vi "CRYReplace Acquisition Curve Name.vi"(6 "Calibration in":string, 7 "Setup in":T3={"No.VI"=0, "Category"="", "StepName"="", "Seq setup flattened"="", "Comment"="", "Steps config."=[], "Jump config"=[], "Start"=0.0, "Increment"=0.0, "Name"="Pa", "Unit"="Pa", "Y data"=1, "Y prefix"="", "Y dB ref"=1.0, "Y unit"="", "Repeat State Array"=[]} {"Repeat State Array"."Start" format="%#_5g"; "Y dB ref" format="%.1f"; "Y data" items=["dB", "Lin"]; "Start" format="%#_5g"}, 8 "Hardware Setup In":string, 9 "Step Setup In":string, 10 "No Insert CurveLib?":bool, 11 "Type In":string) -> (0 "Current Name Out":string[][](array[string]), 2 "Waves Out":T2 {"Y dB ref" format="%.1f"; "Y axis" items=["Log", "Lin"]; "Y data" items=["dB", "Lin"]; "X data" items=["dB", "Lin"]}, 3 "Inserted Names Out":string[](array[string]))   [LabVIEW 2013]
uses:
  Typedef Control/CRYData Variant Array.ctl
  Typedef Control/CRYWaveform Cluster.ctl
  Typedef Control/CRYData Cluster.ctl
  Typedef Control/CRYStep.ctl
  Typedef Control/CRYWaveform Cluster Array.ctl
  Calibration/SubVI/CRYCal Global.vi
panel:
  out "Index for testinfor":i32
  in  "Waveform Cluster":T1={"Waveform"={"X0"=0.0, "dX"=0.0, "Y"=[]}, "X data"=1, "Y data"=1, "Y axis"=1, "X unit"="s", "Y unit"="V", "Y dB ref"=1.0, "display Y"=TRUE, "display X"=TRUE, "Overload?"=FALSE, "Test Info"="", "Step No."=0, "Name"="", "protected"=FALSE, "Sqc history"=[], "Signal Channel ID"=0, "Plot Settings"={"Color"=0, "Interpolation"=0, "Point Style"=0, "Line Style"=0, "Point Color"=0, "Line Width"=0, "Bar Plot Style"=0, "Fill To"=0}, "AutoProtect"=FALSE} {"Y dB ref" format="%.1f"; "Y axis" items=["Log", "Lin"]; "Y data" items=["dB", "Lin"]; "X data" items=["dB", "Lin"]}
  in  "Data In":T4[](array[typedef]) {"Z data" items=["dB", "Lin"]; "X data" items=["dB", "Lin"]; "Y data" items=["dB", "Lin"]; "Z dB ref" format="%.1f"; "Z axis" items=["Log", "Lin"]; "X dB ref" format="%.1f"; "X axis" items=["Log", "Lin"]; "Y axis" items=["Log", "Lin"]; "Y dB ref" format="%.1f"; "Curve"."z" format="%.2f"; "Curve"."y" format="%.2f"; "Curve"."x" format="%.2f"}
  in  "Wave In":T1[](array[typedef]) {"Y dB ref" format="%.1f"; "Y axis" items=["Log", "Lin"]; "Y data" items=["dB", "Lin"]; "X data" items=["dB", "Lin"]}
  in  "Data":T5
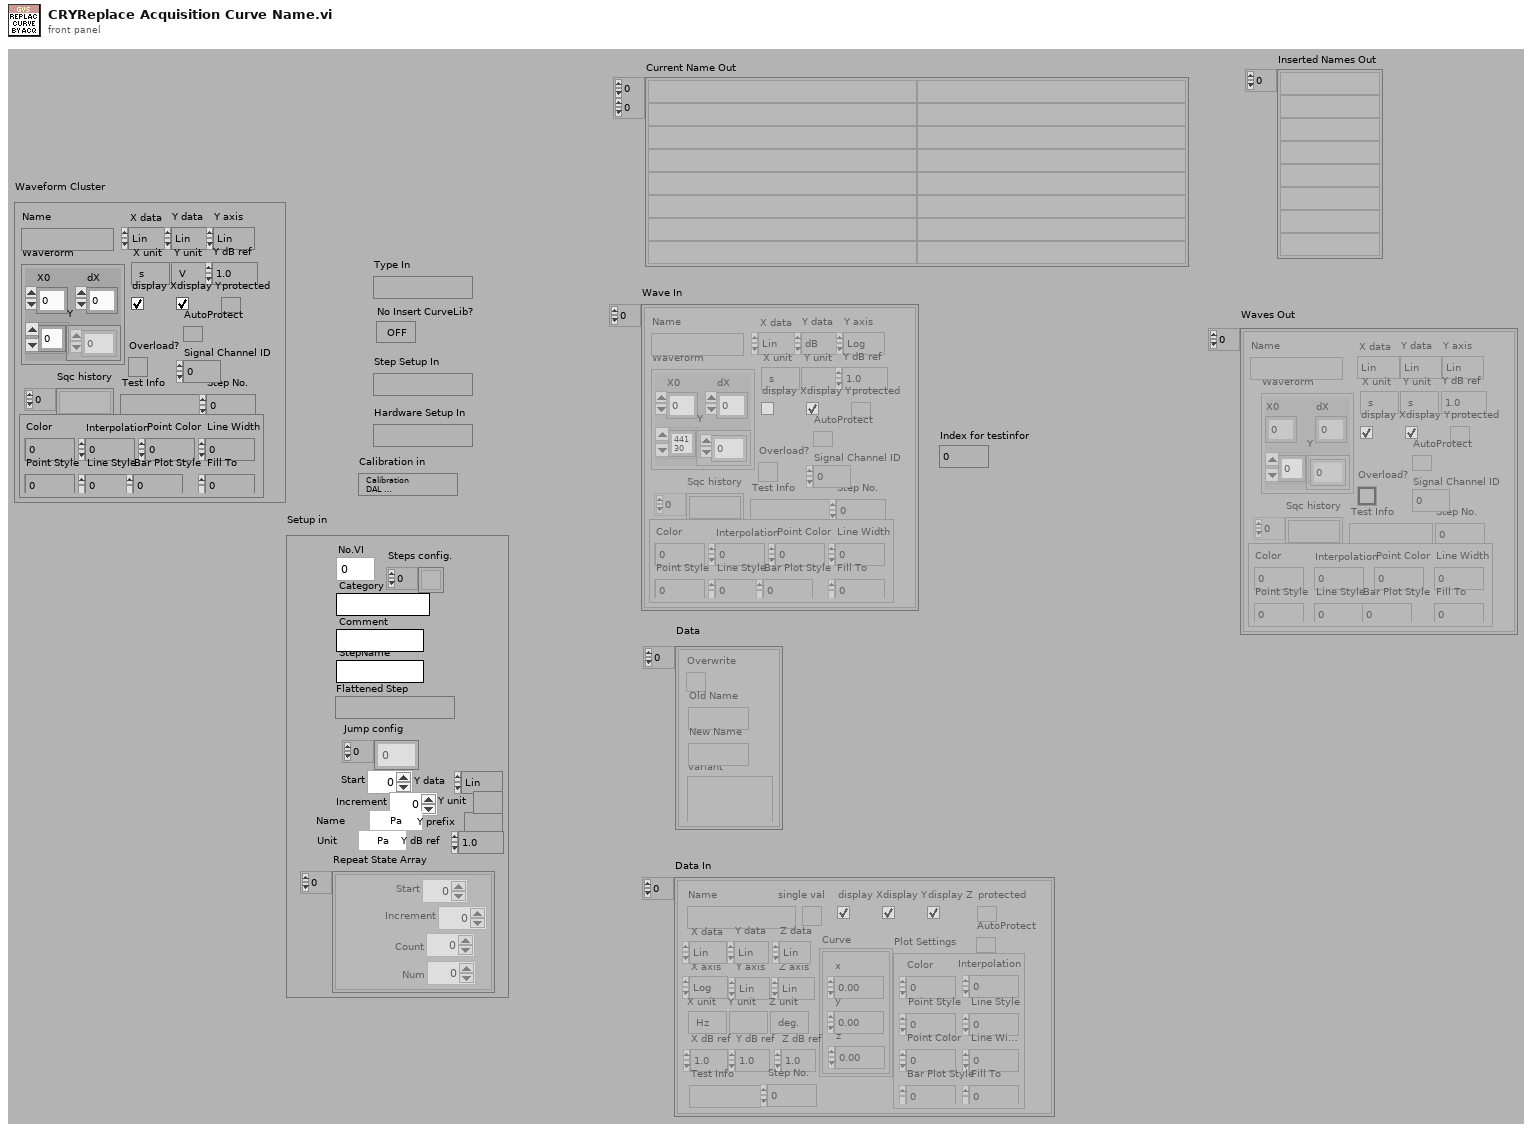
[diagram p1: front panel]
types:
  T1 = typedef "CRYWaveform Cluster.ctl" = cluster{"Waveform":cluster{"X0":dbl, "dX":dbl, "Y":sgl[]}, "X data":u16, "Y data":u16, "Y axis":u16, "X unit":string, "Y unit":string, "Y dB ref":dbl, "display Y":bool, "display X":bool, "Overload?":bool, "Test Info":string, "Step No.":i32, "Name":string, "protected":bool, "Sqc history":string[], "Signal Channel ID":i32, "Plot Settings":cluster{"Color":u32, "Interpolation":u8, "Point Style":u8, "Line Style":u8, "Point Color":u32, "Line Width":u8, "Bar Plot Style":u8, "Fill To":i16}, "AutoProtect":bool}
  T2 = typedef "CRYWaveform Cluster Array.ctl" = T1[]
  T3 = typedef "CRYStep.ctl" = cluster{"No.VI":i32, "Category":string, "StepName":string, "Seq setup flattened":string, "Comment":string, "Steps config.":bool[], "Jump config":i32[], "Start":dbl, "Increment":dbl, "Name":string, "Unit":string, "Y data":u16, "Y prefix":string, "Y dB ref":dbl, "Y unit":string, "Repeat State Array":cluster{"Start":dbl, "Increment":dbl, "Count":i32, "Num":i32}[]}
  T4 = typedef "CRYData Cluster.ctl" = cluster{"Name":string, "Curve":cluster{"x":dbl, "y":dbl, "z":dbl}[], "X data":u16, "Y data":u16, "Z data":u16, "X axis":u16, "Y axis":u16, "Z axis":u16, "X unit":string, "Y unit":string, "Z unit":string, "X dB ref":dbl, "Y dB ref":dbl, "Z dB ref":dbl, "single val":bool, "protected":bool, "display X":bool, "display Y":bool, "display Z":bool, "Test Info":string, "Step No.":i32, "Plot Settings":cluster{"Color":u32, "Interpolation":u8, "Point Style":u8, "Line Style":u8, "Point Color":u32, "Line Width":u8, "Bar Plot Style":u8, "Fill To":i16}, "AutoProtect":bool}
  T5 = typedef "CRYData Variant Array.ctl" = cluster{"variant":variant, "Overwrite":bool, "Old Name":string, "New Name":string}[]
  T6 = enum16{"Play & Record", "Record", "Sine Generator", "Voltmeter", "Oscilloscope", "Spectrum Analyzer", "RTA", "Generator & Voltmeter", "Generator & Oscilloscope", "Generator & Spectrum", "Generator & RTA"}
  T7 = typedef "CRYAcquisition Cluster.ctl" = cluster{"Mode":u16, "Name":string, "use ch name":bool, "Record Time":dbl, "hide rec":bool, "hide play":bool, "rec delay":dbl, "rec pad":dbl, "dcc units":i8, "sine gen setting":string, "scope_fft setting":string, "voltmeter setting":string, "rta setting":string, "trig offset(sec)":dbl, "triggered  record":bool, "trig level":dbl, "trig unit":u8, "trig slop":bool, "trig timeout(sec)":dbl, "add record":bool, "EQ":bool, "record table":string[][], "play table":string[][], "trig channel":string, "Help":string}
  T8 = cluster{"Start":dbl, "Increment":dbl, "Count":i32, "Num":i32}[]
  T9 = typedef "CRYCalibration 2DCluster.ctl" = cluster{"Calibration":T10, "Corr Curve":T4, "EQ Curve":T4, "Sens Curve":T4}
  T10 = typedef "CRYCalibration Cluster.ctl" = cluster{"Calibration Step Name":string, "Device":string, "Correction Curve Name":string, "Equalization Curve Name":string, "Sensitivity Curve Name":string, "Corr Folder and File":string, "EQ Folder and File":string, "Sens Folder and File":string, "Corr Step size":u16, "EQ Step size":u16, "Input":bool, "Last Cal Date (sec)":timestamp, "Cha Name":string, "Corr Curve Found":bool, "EQ Curve Found":bool, "Sens Curve Found":bool, "Signal Type":string, "Calibrated Device":string, "Hz":u32}
  T11 = typedef "CRYCalibration All Cluster.ctl" = cluster{"Calibration 2D":T9[], "Help":string, "Tab Value":i32, "Input Signal Type":string, "Output Signal Type":string}
  T12 = typedef "CRYHardware Channel Info.ctl" = cluster{"ID":i32, "Name":string, "Digital":bool, "Input":bool, "Device Name":string, "Hardware Ch ID":u8, "Vmax (V)":dbl, "Latency (samples)":dbl, "Sampling Rate (Hz)":u32, "Bit Depth":u32, "Anti-aliasing Factor (%fs)":sgl, "DAQmx Channel":tag, "term config":i32, "Coupling":i32, "IEPE en":bool, "ASIOChannel Name":string, "Audio Driver":u16, "ASIOChannel Index":u8}
  T13 = cluster{"MME Record Cluster":cluster{"RecDeviceID":u32, "RecSampleFreq":u32, "RecChannels":u32, "RecBitDepth":u32, "RecSampleData":i32[], "RecDataLength":u32, "RecTime":sgl, "RecLatency":sgl, "RecPadding":sgl, "nBufferUse":u32, "nRealTime":u32, "Anti Alias":u32, "Device Name":string, "Audio Driver":u16}[], "ASIO Record Cluster":cluster{"RecDeviceID":u32, "RecSampleFreq":u32, "RecChannels":u32, "RecBitDepth":u32, "RecSampleData":i32[], "RecDataLength":u32, "RecTime":sgl, "RecLatency":sgl, "RecPadding":sgl, "nBufferUse":u32, "nRealTime":u32, "Anti Alias":u32, "Device Name":string, "Audio Driver":u16}[]}
  T14 = cluster{"RecDeviceID":u32, "RecSampleFreq":u32, "RecChannels":u32, "RecBitDepth":u32, "RecSampleData":i32[], "RecDataLength":u32, "RecTime":sgl, "RecLatency":sgl, "RecPadding":sgl, "nBufferUse":u32, "nRealTime":u32, "Anti Alias":u32, "Device Name":string, "Audio Driver":u16}[]
  T15 = typedef "CRYStimulus Test Infor Cluster.ctl" = cluster{"Stimulus Type":string, "Signal Type":string, "In/Out":bool, "FAPS":cluster{"freq":dbl, "ampl":dbl, "cycles":dbl, "samples":i32}[], "Sampling Rate":dbl, "Samples":i32, "Analysis Param":string, "Resolution":u16, "Steps":u32, "Analysis Value":dbl[], "Diff Freq":dbl, "FStart":dbl, "FStop":dbl, "Calibration Param":string, "Anti Alias":dbl, "Level Out1":dbl, "Level Out2":dbl, "EQ":bool}
  T16 = typedef "CRYData Cluster Array.ctl" = T4[]
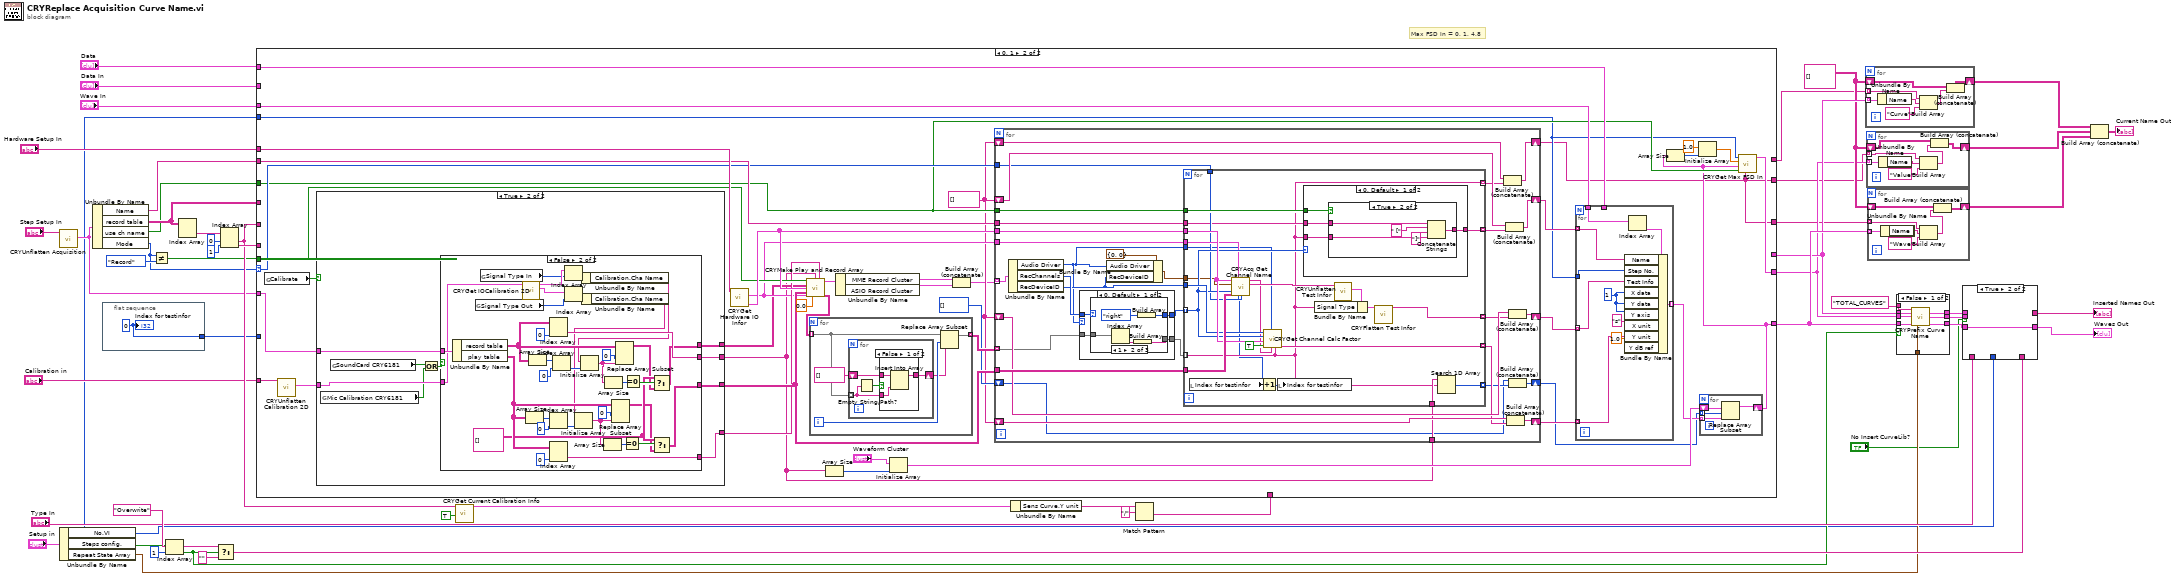
[diagram p0: block diagram]
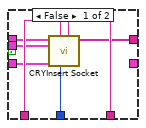
[diagram p2: hidden frame]
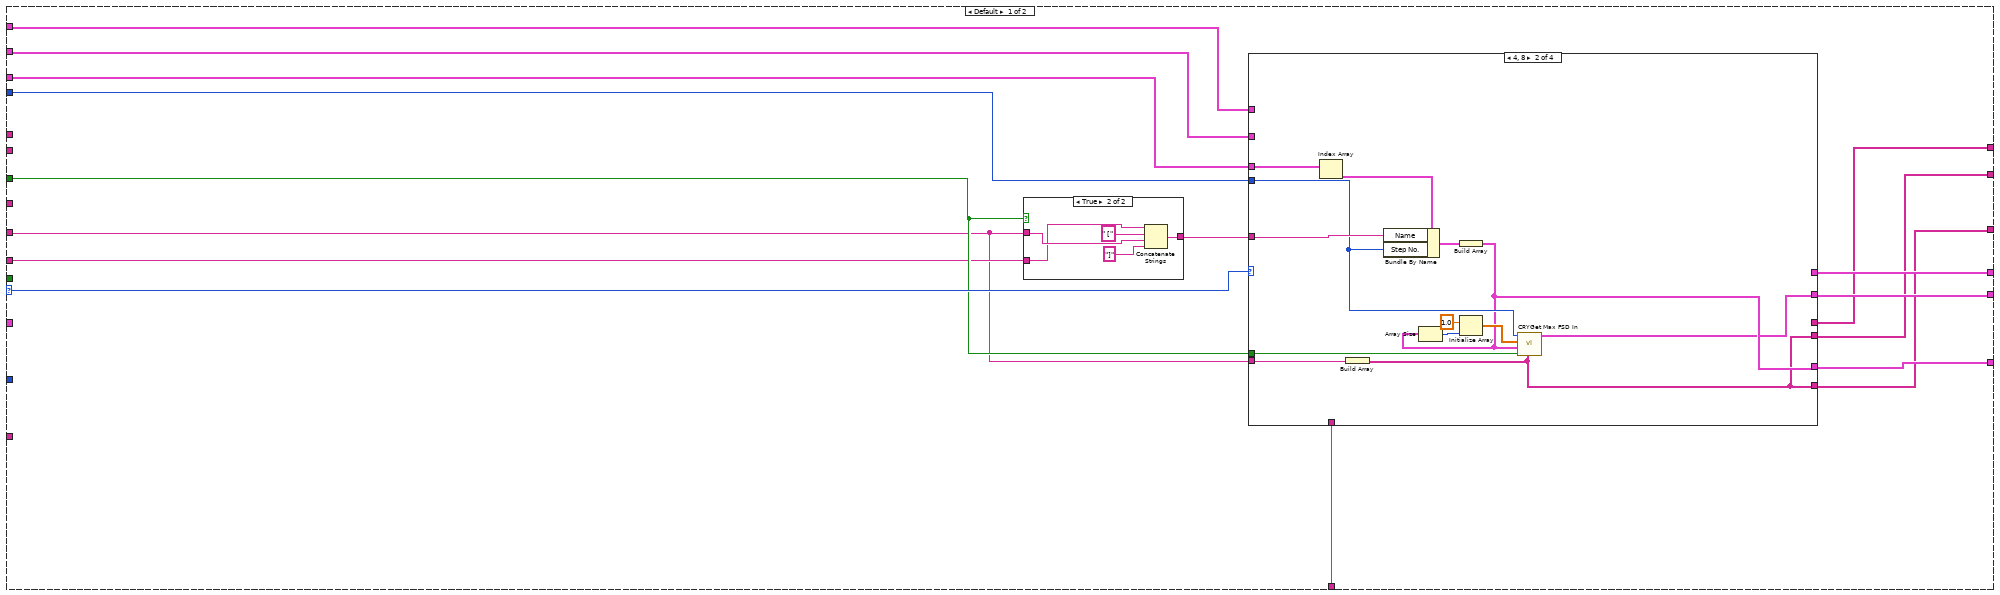
[diagram p4: hidden frame]
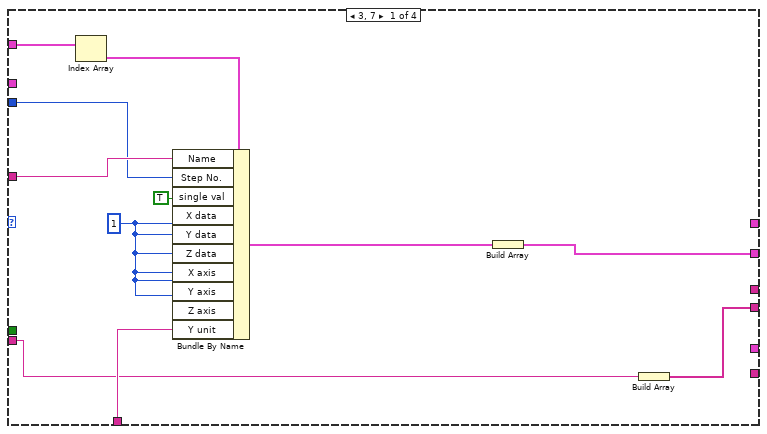
[diagram p5: hidden frame]
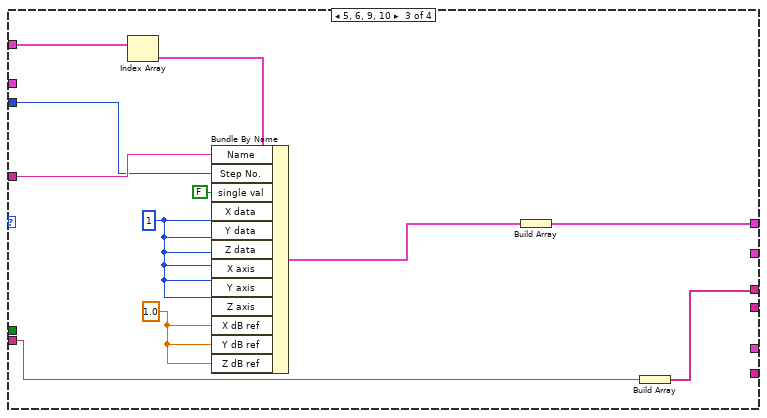
[diagram p6: hidden frame]
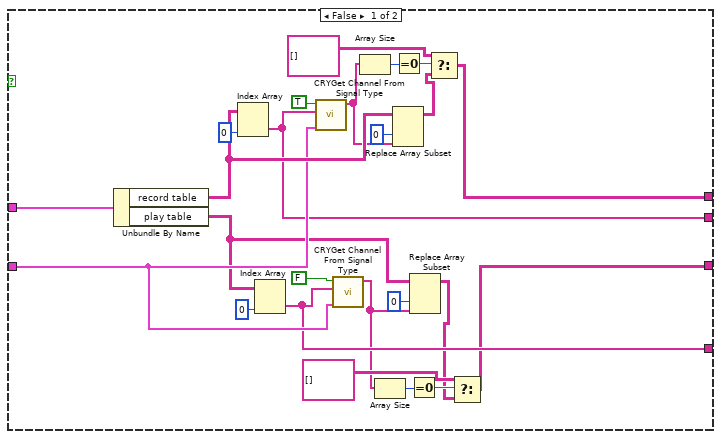
[diagram p10: hidden frame]
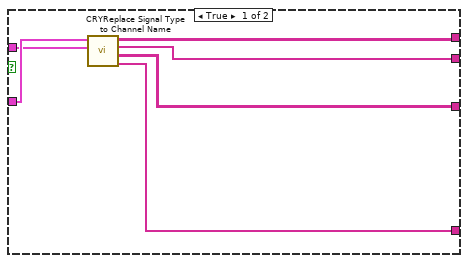
[diagram p11: hidden frame]
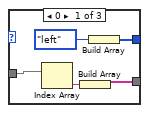
[diagram p12: hidden frame]
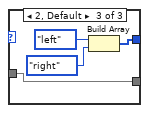
[diagram p13: hidden frame]
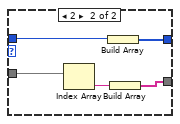
[diagram p14: hidden frame]
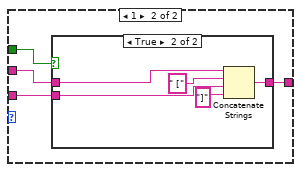
[diagram p16: hidden frame]
diagram:
  w11 = string[][] []
  # "Max FSD In = 0, 1, 4,8"
  n1 = call "CRYUnflatten Acquisition.vi"("Flatten Acquisition"="Step Setup In") -> ("Acquisition"=w17:T7)  [unwired: 10 out]
  n2 = Unbundle By Name("Setup in") -> ("No.VI"=w14:i32, "Steps config."=w33:bool[], "Repeat State Array"=w24:T8)
  n3 = Unbundle By Name(w17) -> ("Name"=w16:string, "record table"=w20:string[][], "use ch name"=w10:bool, "Mode"=w15:u16)
  n4 = flat-sequence {
    tunnel: [w53] -> w1
    frame #0 {
      w53 = 0 ("Index for testinfor")
      "Index for testinfor" <- w53
    }
  }
  n5 = Not Equal?(x=w15, y=T6."Record" ("Record Mode")) -> (x != y?=w19:bool)
  n6 = Index Array(array=w33, index=1) -> (element=w25:bool)
  n7 = Index Array(array=w20) -> (element=w48:string[])  [unwired: 2 in]
  n8 = Select(t="Overwrite" ("Y unit"), s=w25, f="") -> (s? t:f=w31:string)
  n9 = Index Array(array=w48, index #1=0 ("index"), index #2=1 ("index")) -> (element #1=w39:string, element #2=w47:string)
  n10 = call "CRYGet Current Calibration Info.vi"("Is Input?"=TRUE, "Signal Type Name"=w39) -> ("Calibration All Cluster"=w42:T9)  [unwired: 9 out]
  n11 = Unbundle By Name(w42) -> ("Sens Curve.Y unit"=w40:string)
  n12 = Match Pattern(string=w40, regular expression="/" ("search char (-)")) -> (after substring=w38:string)  [unwired: 4 out]
  n13 = case shown="0, 1" w15 {
    selector: w15 -> [w64 w134]
    tunnel: w47 -> [w58 _]
    tunnel: w10 -> [w59 w120]
    tunnel: w39 -> [w57 _]
    tunnel: "Data" -> [w68 w149]
    tunnel: "Wave In" -> [w67 w148]
    tunnel: w14 -> [w65 w118]
    tunnel: "Data In" -> [w69 _]
    tunnel: w38 -> [w63 _]
    tunnel: [w61 w117] -> w13
    tunnel: [w62 w119] -> w9
    tunnel: [w60 _] -> w12
    tunnel: "Hardware Setup In" -> [_ w145]
    tunnel: w20 -> [_ _]
    tunnel: w19 -> [_ w143]
    tunnel: "Calibration in" -> [_ w141]
    tunnel: w17 -> [_ w140]
    tunnel: w16 -> [_ w135]
    tunnel: [w54 w115] -> w4
    tunnel: [w56 w115] -> w3
    tunnel: [w55 _] -> w2
    tunnel: w1 -> [_ _]
    frame Default {
      n14 = case shown="True" w59 {
        tunnel: w57 -> [_ w108]
        tunnel: [w105 w107] -> w66
        tunnel: w58 -> [w105 w106]
        frame False {
        }
        frame True {
          n15 = Concatenate Strings(w106, " [" ("string"), w108, "]" ("string")) -> (w107:string)
        }
      }
      n16 = case shown="4, 8" w64 {
        tunnel: w67 -> [_ w93 _ _]
        tunnel: w68 -> [_ _ _ _]
        tunnel: w69 -> [w80 _ w104 _]
        tunnel: w66 -> [w78 w91 w102 _]
        tunnel: w65 -> [w74 w85 w98 _]
        tunnel: w63 -> [w75 _ _ _]
        tunnel: [w72 w83 _ _] -> w62
        tunnel: [_ w84 _ _] -> w61
        tunnel: [_ _ w96 _] -> w60
        tunnel: w59 -> [_ w86 _ _]
        tunnel: w57 -> [w71 w82 w95 _]
        tunnel: [_ w81 _ _] -> w56
        tunnel: [_ _ w94 _] -> w55
        tunnel: [w70 w81 _ _] -> w54
        frame 3, 7 {
          w76 = u16 1 ("X data")
          n17 = Index Array(array=w80) -> (element=w79:T4)  [unwired: 1 in]
          n18 = Bundle By Name(cluster=w79, "Name"=w78, "Step No."=w74, "single val"=TRUE, "X data"=w76, "Y data"=w76, "Z data"=w76, "X axis"=w76, "Y axis"=w76, "Z axis"=w76, "Y unit"=w75) -> (w73:T4)
          n19 = Build Array(w73) -> (w72:T4[])
          n20 = Build Array(w71) -> (w70:string[])
        }
        frame 4, 8 {
          n21 = Index Array(array=w93) -> (element=w92:T1)  [unwired: 1 in]
          n22 = Build Array(w82) -> (w81:string[])
          n23 = Bundle By Name(cluster=w92, "Name"=w91, "Step No."=w85) -> (w90:T1)
          n24 = Build Array(w90) -> (w84:T1[])
          n25 = Array Size(array=w84) -> (size(s)=w87:i32)
          n26 = Initialize Array(1.0 ("element"), w87) -> (w89:dbl[])
          n27 = call "CRYGet Max FSD In.vi"("Signal Path"=w81, "use ch name"=w86, "Wave in"=w84, "Max Level"=w89, "Step No."=w85) -> ("Data Out"=w83:T4[])  [unwired: 6 in]
        }
        frame 5, 6, 9, 10 {
          w99 = 1.0 ("X dB ref")
          w100 = u16 1 ("X data")
          n28 = Index Array(array=w104) -> (element=w103:T4)  [unwired: 1 in]
          n29 = Bundle By Name(cluster=w103, "Name"=w102, "Step No."=w98, "single val"=FALSE, "X data"=w100, "Y data"=w100, "Z data"=w100, "X axis"=w100, "Y axis"=w100, "Z axis"=w100, "X dB ref"=w99, "Y dB ref"=w99, "Z dB ref"=w99) -> (w97:T4)
          n30 = Build Array(w97) -> (w96:T4[])
          n31 = Build Array(w95) -> (w94:string[])
        }
        frame Default {
        }
      }
    }
    frame 0, 1 {
      w116 = string[] [] ("appended array")
      n32 = global read "CRYCal Global.vi" "Calibrate"() -> (w139:bool)
      n33 = call "CRYUnflatten Calibration 2D.vi"("Flattened Calibration"=w141) -> ("Calibration Step Out"=w142:T11)  [unwired: 8 in, 2 out]
      n34 = case shown="True" w139 {
        tunnel: [w175 w197] -> w130
        tunnel: [w169 w196] -> w138
        tunnel: w140 -> [w192 w201]
        tunnel: w142 -> [w184 w198]
        tunnel: [w182 w200] -> w137
        tunnel: [w181 w199] -> w126
        frame False {
          n35 = Unbundle By Name(w192) -> ("record table"=w189:string[][], "play table"=w183:string[][])
          n36 = Index Array(array=w189, index (col)=0 ("disabled index (col)")) -> (element=w181:string[])  [unwired: 1 in]
          n37 = Index Array(array=w183, index (col)=0 ("disabled index (col)")) -> (element=w182:string[])  [unwired: 1 in]
          n38 = call "CRYGet Channel From Signal Type.vi"("Calibration"=w184, "Signal Type Name Array In"=w181, "In/Out?"=TRUE) -> ("Channel Name Array Out"=w177:string[])  [unwired: 7 in, 1 out]
          n39 = call "CRYGet Channel From Signal Type.vi"("Calibration"=w184, "Signal Type Name Array In"=w182, "In/Out?"=FALSE) -> ("Channel Name Array Out"=w171:string[])  [unwired: 7 in, 1 out]
          n40 = Array Size(array=w177) -> (size(s)=w178:i32)
          n41 = Array Size(array=w171) -> (size(s)=w174:i32)
          n42 = Replace Array Subset(array=w189, new element=w177, index (col)=0 ("disabled index (col)")) -> (w176:string[][])  [unwired: 1 in]
          n43 = Equal To 0?(x=w178) -> (x = 0?=w179:bool)
          n44 = Equal To 0?(x=w174) -> (x = 0?=w173:bool)
          n45 = Replace Array Subset(array=w183, new element=w171, index (col)=0 ("disabled index (col)")) -> (w170:string[][])  [unwired: 1 in]
          n46 = Select(t=string[][] [] ("output array"), s=w179, f=w176) -> (s? t:f=w175:string[][])
          n47 = Select(t=string[][] [] ("output array"), s=w173, f=w170) -> (s? t:f=w169:string[][])
        }
        frame True {
          n48 = global read "CRYCal Global.vi" "Mic Calibration CRY6181"() -> (w195:bool)
          n49 = global read "CRYCal Global.vi" "SoundCard CRY6181"() -> (w194:bool)
          n50 = Or(x=w194, y=w195) -> (x .or. y?=w193:bool)
          n51 = case shown="False" w193 {
            tunnel: w201 -> [w206 w239]
            tunnel: [w202 w231] -> w200
            tunnel: [w204 w228] -> w199
            tunnel: w198 -> [w207 w227]
            tunnel: [w203 w211] -> w196
            tunnel: [w205 w208] -> w197
            frame True {
              n52 = call "CRYReplace Signal Type to Channel Name.vi"("Acquisition step in"=w206, "Calibration Step in"=w207) -> ("Play Signal Type"=w202:string[], "Play table"=w203:string[][], "Record Signal Type"=w204:string[], "record table"=w205:string[][])  [unwired: 6 in]
            }
            frame False {
              w213 = string[][] [] ("output array")
              n53 = Unbundle By Name(w239) -> ("record table"=w229:string[][], "play table"=w233:string[][])
              n54 = global read "CRYCal Global.vi" "Signal Type Out"() -> (w219:u16)
              n55 = global read "CRYCal Global.vi" "Signal Type In"() -> (w223:u16)
              n56 = call "CRYGet IOCalibration 2D.vi"("Calibration"=w227) -> ("O_Calibration 2D Out"=w220:T9[], "I_Calibration 2D Out"=w224:T9[])  [unwired: 9 in]
              n57 = Array Size(array=w233) -> (size(s)=w234:i32[])
              n58 = Array Size(array=w229) -> (size(s)=w242:i32[])
              n59 = Index Array(array=w229, index (col)=0 ("disabled index (col)")) -> (element=w228:string[])  [unwired: 1 in]
              n60 = Index Array(array=w233, index (col)=0 ("disabled index (col)")) -> (element=w231:string[])  [unwired: 1 in]
              n61 = Index Array(array=w234, index=0) -> (element=w237:i32)
              n62 = Index Array(array=w242, index=0) -> (element=w238:i32)
              n63 = Index Array(array=w224, index=w223) -> (element=w222:T9)
              n64 = Index Array(array=w220, index=w219) -> (element=w221:T9)
              n65 = Unbundle By Name(w222) -> ("Calibration.Cha Name"=w226:string)
              n66 = Initialize Array(w226, w238) -> (w214:string[])
              n67 = Unbundle By Name(w221) -> ("Calibration.Cha Name"=w225:string)
              n68 = Initialize Array(w225, w237) -> (w210:string[])
              n69 = Array Size(array=w210) -> (size(s)=w218:i32)
              n70 = Array Size(array=w214) -> (size(s)=w216:i32)
              n71 = Replace Array Subset(array=w233, new element=w210, index (col)=0 ("disabled index (col)")) -> (w212:string[][])  [unwired: 1 in]
              n72 = Replace Array Subset(array=w229, new element=w214, index (col)=0 ("disabled index (col)")) -> (w209:string[][])  [unwired: 1 in]
              n73 = Equal To 0?(x=w218) -> (x = 0?=w217:bool)
              n74 = Equal To 0?(x=w216) -> (x = 0?=w215:bool)
              n75 = Select(t=w213, s=w215, f=w209) -> (s? t:f=w208:string[][])
              n76 = Select(t=w213, s=w217, f=w212) -> (s? t:f=w211:string[][])
            }
          }
        }
      }
      n77 = call "CRYGet Hardware IO Infor.vi"("Hardware setup In"=w145) -> ("I_channel Info Out"=w144:T12[], "O_channel Info Out"=w136:T12[])  [unwired: 9 out]
      n78 = call "CRYMake Play and Record Array.vi"("Play&Record/Record"=w143, "Selected Record Signal Path In"=w126, "Selected Play Signal Path In"=w137, "Selected Record In"=w130, "input channel Info In"=w144, "Selected Play In"=w138, "output channel Info In"=w136, "Rec Time"=0.0) -> ("Record Cluster Out"=w114:T13, "Record Name Array"=w133:string[][])  [unwired: 2 in, 4 out]
      n79 = for {
        tunnel: w133 -> [w159] mode=indexing
        tunnel: [w158] -> w132 mode=indexing
        i -> [w157]
        n80 = for {
          tunnel: w159 -> [w162] mode=indexing
          shift-right: [w161] -> w156
          shift-left: string[] [] ("Record Name Array") -> [w163]
          n81 = Empty String/Path?(string/path=w162) -> (empty?=w164:bool)
          n82 = case shown="False" w164 {
            tunnel: w163 -> [w167 w168]
            tunnel: w162 -> [w166 _]
            tunnel: [w165 w168] -> w161
            frame False {
              n83 = Insert Into Array(array=w167, new element=w166) -> (w165:string[])  [unwired: 1 in]
            }
            frame True {
            }
          }
        }
        n84 = Replace Array Subset(array=w159, new element=w156, index=w157) -> (w158:string[])
      }
      n85 = Array Size(array=w126) -> (size(s)=w131:i32)
      n86 = Unbundle By Name(w114) -> ("MME Record Cluster"=w113:T14, "ASIO Record Cluster"=w112:T14)
      n87 = Initialize Array("Waveform Cluster", w131) -> (w128:T1[])
      n88 = Build Array (concatenate)(w113, w112) -> (w111:T14)
      n89 = for {
        tunnel: w111 -> [w283] mode=indexing
        tunnel: w144 -> [w280]
        tunnel: w138 -> [w279]
        tunnel: w120 -> [w278]
        tunnel: w135 -> [w277]
        shift-right: [w274] -> w151
        shift-left: w116 -> [w275]
        shift-right: [w271] -> w150
        shift-left: w116 -> [w273]
        shift-right: [w268] -> w147
        shift-left: w116 -> [w270]
        tunnel: w132 -> [w267] mode=indexing
        tunnel: w136 -> [w265]
        tunnel: w134 -> [w264]
        tunnel: w126 -> [w263]
        shift-right: [w261] -> w124
        shift-left: i32[] [] -> [w260]
        shift-right: [w257] -> w115
        shift-left: w116 -> [w258]
        n90 = Unbundle By Name(w283) -> ("Audio Driver"=w253:u16, "RecChannels"=w282:u32, "RecDeviceID"=w255:u32)
        n91 = case shown="0, Default" w253 {
          tunnel: w282 -> [w287 w302]
          tunnel: [w286 w306] -> w281
          tunnel: w267 -> [w285 w305]
          tunnel: [w284 w304] -> w266
          frame 0, Default {
            n92 = case shown="1" w287 {
              tunnel: [w291 w296 w299] -> w286
              tunnel: w285 -> [w289 w294 w298]
              tunnel: [w288 w293 w298] -> w284
              frame 0 {
                n93 = Index Array(array=w289) -> (element=w290:string)  [unwired: 1 in]
                n94 = Build Array(w290) -> (w288:string[])
                n95 = Build Array(enum16{"left", "right"}."left") -> (w291:enum16{"left", "right"}[])
              }
              frame 1 {
                n96 = Index Array(array=w294) -> (element=w295:string)  [unwired: 1 in]
                n97 = Build Array(w295) -> (w293:string[])
                n98 = Build Array(enum16{"left", "right"}."right") -> (w296:enum16{"left", "right"}[])
              }
              frame 2, Default {
                n99 = Build Array(enum16{"left", "right"}."left", enum16{"left", "right"}."right") -> (w299:enum16{"left", "right"}[])
              }
            }
          }
          frame 2 {
            n100 = Index Array(array=w305) -> (element=w303:string)  [unwired: 1 in]
            n101 = Build Array(w302) -> (w306:u32[])
            n102 = Build Array(w303) -> (w304:string[])
          }
        }
        n103 = Bundle By Name(cluster=cluster{"RecDeviceID":u32, "Audio Driver":u32} {"RecDeviceID"=0, "Audio Driver"=0} ("Cluster"), "Audio Driver"=w253, "RecDeviceID"=w255) -> (w254:cluster{"RecDeviceID":u32, "Audio Driver":u32})
        n104 = for {
          tunnel: w281 -> [w320] mode=indexing
          tunnel: w255 -> [w321]
          tunnel: w280 -> [w322]
          tunnel: w279 -> [w329]
          tunnel: w278 -> [w325]
          tunnel: w277 -> [w312]
          tunnel: [w324] -> w276 mode=indexing
          tunnel: [w323] -> w272 mode=indexing
          tunnel: [w318] -> w269 mode=indexing
          tunnel: w266 -> [w311] mode=indexing
          tunnel: w265 -> [w316]
          tunnel: w264 -> [w315]
          tunnel: w263 -> [w314]
          tunnel: [w313] -> w262 mode=indexing
          tunnel: [w311] -> w259 mode=indexing
          tunnel: w254 -> [w310]
          tunnel: w253 -> [w309]
          n105 = local read "Index for testinfor"() -> (w307:i32)
          n106 = call "CRYAcq Get Channel Name.vi"("I_channel Info Out"=w322, "O_channel Info Out"=w316, "Cluster"=w310, "RecChannel"=w320, "Selected Play In"=w329, "Index for testinfor"=w307, "Acquisition Type"=w315) -> ("ChannelName In"=w317:string, "Test Info"=w326:string)  [unwired: 3 in, 4 out]
          n107 = Increment(x=w307) -> (x+1=w308:i32)
          n108 = call "CRYGet Channel Calc Factor.vi"("Signal Path"=w311, "Channel Name"=w317, "Audio Driver"=w309, "Is Input?"=TRUE, "I/O_channel Info"=w322, "Channel(LR)"=w320, "DeviceID"=w321) -> ("Y unit"=w318:string)  [unwired: 4 out]
          n109 = local write "Index for testinfor"(w308) -> ()
          n110 = case shown="0, Default" w320 {
            tunnel: [w332 w342] -> w324
            tunnel: w312 -> [w333 w343]
            tunnel: w311 -> [w331 w341]
            tunnel: w325 -> [w330 w340]
            frame 0, Default {
              n111 = case shown="True" w330 {
                tunnel: w333 -> [w334 w337]
                tunnel: [w334 w336] -> w332
                tunnel: w331 -> [_ w335]
                frame False {
                }
                frame True {
                  n112 = Concatenate Strings(w337, " [" ("string"), w335, "]" ("string")) -> (w336:string)
                }
              }
            }
            frame 1 {
              n113 = case shown="True" w340 {
                tunnel: w343 -> [w344 w347]
                tunnel: [w344 w346] -> w342
                tunnel: w341 -> [_ w345]
                frame False {
                }
                frame True {
                  n114 = Concatenate Strings(w347, " [" ("string"), w345, "]" ("string")) -> (w346:string)
                }
              }
            }
          }
          n115 = call "CRYUnflatten Test Infor.vi"("Falattend test infor"=w326) -> ("unflattened test infor data"=w328:T15)  [unwired: 9 out]
          n116 = Bundle By Name(cluster=w328, "Signal Type"=w311) -> (w327:T15)
          n117 = call "CRYFlatten Test Infor.vi"("Test Infor data"=w327) -> ("Fattened Data"=w323:string)  [unwired: 10 out]
          n118 = Search 1D Array(1D array=w314, element=w311) -> (index of element=w313:i32)  [unwired: 1 in]
        }
        n119 = Build Array (concatenate)(w258, w259) -> (w257:string[])
        n120 = Build Array (concatenate)(w275, w276) -> (w274:string[])
        n121 = Build Array (concatenate)(w270, w269) -> (w268:string[])
        n122 = Build Array (concatenate)(w273, w272) -> (w271:string[])
        n123 = Build Array (concatenate)(w260, w262) -> (w261:i32[])
      }
      n124 = for {
        tunnel: w151 -> [w243] mode=indexing
        tunnel: w150 -> [w250] mode=indexing
        tunnel: w118 -> [w251]
        tunnel: [w244] -> w127 mode=indexing
        tunnel: w149 -> [_]
        tunnel: w148 -> [w249]
        tunnel: w147 -> [w245] mode=indexing
        w248 = u16 1 ("X data")
        n125 = Index Array(array=w249) -> (element=w252:T1)  [unwired: 1 in]
        n126 = Bundle By Name(cluster=w252, "Name"=w243, "Step No."=w251, "Test Info"=w250, "X data"=w248, "Y data"=w248, "Y axis"=w248, "X unit"="s", "Y unit"=w245, "Y dB ref"=1.0) -> (w244:T1)
      }
      n127 = for {
        tunnel: w124 -> [w154] mode=indexing
        tunnel: w127 -> [w153] mode=indexing
        shift-right: [w152] -> w117
        shift-left: w128 -> [w155]
        n128 = Replace Array Subset(array=w155, new element=w153, index=w154) -> (w152:T1[])
      }
      n129 = Array Size(array=w117) -> (size(s)=w121:i32)
      n130 = Initialize Array(1.0 ("element"), w121) -> (w123:dbl[])
      n131 = call "CRYGet Max FSD In.vi"("Signal Path"=w115, "use ch name"=w120, "Wave in"=w117, "Max Level"=w123, "Step No."=w118) -> ("Data Out"=w119:T4[])  [unwired: 6 in]
    }
  }
  n132 = for {
    tunnel: w12 -> [w356] mode=indexing
    shift-right: [w354] -> w8
    shift-left: w11 -> [w355]
    tunnel: w2 -> [w350] mode=indexing
    n133 = Unbundle By Name(w356) -> ("Name"=w353:string)
    n134 = Build Array(w350, w353, "Curve" ("Name")) -> (w351:string[])
    n135 = Build Array (concatenate)(w355, w351) -> (w354:string[][])
  }
  n136 = for {
    tunnel: w9 -> [w363] mode=indexing
    shift-right: [w361] -> w7
    shift-left: w11 -> [w362]
    tunnel: w4 -> [w357] mode=indexing
    n137 = Unbundle By Name(w363) -> ("Name"=w359:string)
    n138 = Build Array(w357, w359, "Value" ("Name")) -> (w358:string[])
    n139 = Build Array (concatenate)(w362, w358) -> (w361:string[][])
  }
  n140 = for {
    tunnel: w13 -> [w370] mode=indexing
    shift-right: [w368] -> w5
    shift-left: w11 -> [w369]
    tunnel: w3 -> [w364] mode=indexing
    n141 = Unbundle By Name(w370) -> ("Name"=w366:string)
    n142 = Build Array(w364, w366, "Wave" ("Name")) -> (w365:string[])
    n143 = Build Array (concatenate)(w369, w365) -> (w368:string[][])
  }
  n144 = case shown="False" w25 {
    tunnel: "TOTAL_CURVES" ("Type In") -> [w378 _]
    tunnel: w12 -> [w377 w381]
    tunnel: w9 -> [w376 w380]
    tunnel: w13 -> [w375 w379]
    tunnel: [w374 w381] -> w28
    tunnel: [w373 w380] -> w27
    tunnel: [w372 w379] -> w26
    tunnel: w24 -> [w371 _]
    frame False {
      n145 = call "CRYPrefix Curve Name.vi"("Type In"=w378, "Curves In"=w377, "Values In"=w376, "Waves In"=w375, "Repeat State Array In"=w371) -> ("Curves Out"=w374:T16, "Values Out"=w373:T16, "Waves Out"=w372:T2)  [unwired: 7 in, 1 out]
    }
    frame True {
    }
  }
  n146 = case shown="True" "No Insert CurveLib?" {
    tunnel: "Type In" -> [w388 _]
    tunnel: w31 -> [w387 _]
    tunnel: [w386 _] -> w30
    tunnel: w28 -> [w385 _]
    tunnel: w27 -> [w384 _]
    tunnel: w26 -> [w383 w389]
    tunnel: w14 -> [w382 _]
    tunnel: [_ w389] -> w22
    frame False {
      n147 = call "CRYInsert Socket.vi"("sOption2"=w387, "Step No."=w382, "sOption1"=w388, "Waves"=w383, "Values"=w384, "Curves"=w385) -> ("Inserted Names Out"=w386:string[])  [unwired: 5 in]
    }
    frame True {
    }
  }
  "Inserted Names Out" <- w30
  "Waves Out" <- w22
  n148 = Build Array (concatenate)(w8, w7, w5) -> (→"Current Name Out":string[][])
